vi "Frame size enum to U32 value.vi"(1 "Value":T1 items=["100X100"=100, "128X128"=128, "200X200"=200, "256X256"=256, "512X512"=512, "1024x1024"=1024, "2048x2048"=2048]) -> (0 "Frame Size U32":u32)   [LabVIEW 2020]
uses:
  Typedefs/Frame Size.ctl
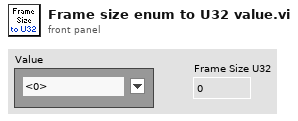
[diagram p1: front panel]
types:
  T1 = typedef "Frame Size.ctl" = u16
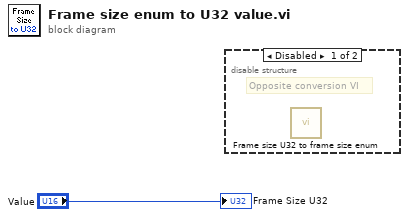
[diagram p0: block diagram]
diagram:
  n1 = disable-structure shown="Disabled" {
    frame Disabled {
      # "Opposite conversion VI"
      n2 = call "Frame size U32 to frame size enum.vi"() -> ()  [unwired: 1 in, 1 out]
    }
    frame Enabled {
    }
  }
  "Frame Size U32" <- "Value"
